vi "setup-reflux.vi"(8 "Reflux Ratio":dbl, 9 "Period (Seconds) in":dbl=5.0, 10 "Sampling Mode":T2(ring), 11 "delaytimes mS in":cluster{"low":dbl, "high":dbl}) -> (0 "Duty %":dbl, 1 "HIGH Cycle Time (Seconds)":dbl, 2 "LOW Cycle Time (Seconds)":dbl, 3 "delaytimes mS out":cluster{"low":dbl, "high":dbl}, 4 "Disabled":T1(ring), 6 "Period (Seconds) out":dbl)   [LabVIEW 2024]
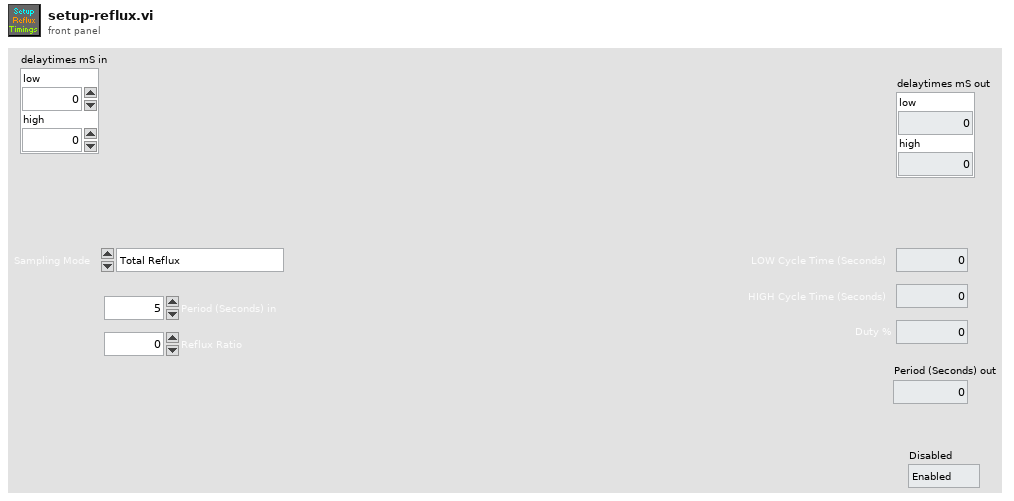
[diagram p1: front panel]
types:
  T1 = enum8{"Enabled", "Disabled", "Disabled and Grayed Out"}
  T2 = enum16{"Total Reflux", "Total Withdrawl", "Reflux Ratio"}
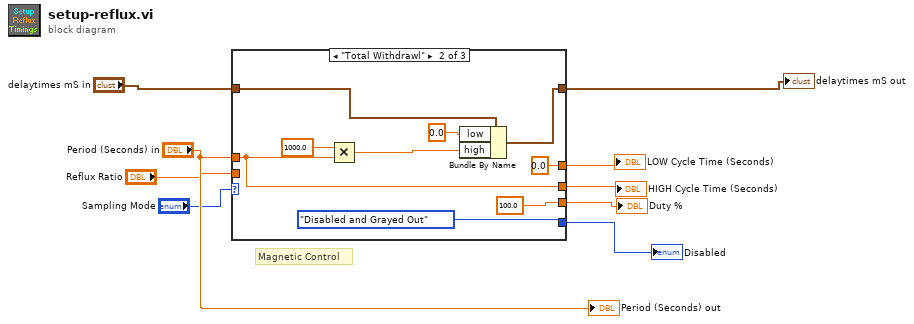
[diagram p0: block diagram]
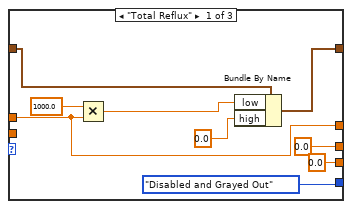
[diagram p2: hidden frame]
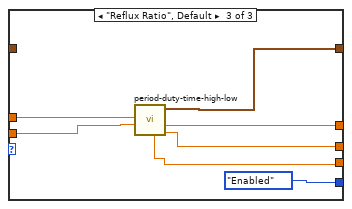
[diagram p3: hidden frame]
diagram:
  # "Magnetic Control"
  n1 = case shown="\"Total Withdrawl\"" "Sampling Mode" {
    tunnel: [w10 w26 w31] -> w4
    tunnel: "Period (Seconds) in" -> [w11 w24 w32]
    tunnel: "Reflux Ratio" -> [_ _ w33]
    tunnel: [w11 0.0 ("Time Low (Seconds)") w30] -> w5
    tunnel: [0.0 ("Time High (Seconds)") w24 w29] -> w6
    tunnel: [0.0 ("Duty %") 100.0 ("Duty %") w28] -> w7
    tunnel: [T1."Disabled and Grayed Out" ("Disabled") T1."Disabled and Grayed Out" ("Disabled") T1."Enabled" ("Disabled")] -> w1
    tunnel: "delaytimes mS in" -> [w18 w27 _]
    frame "Total Reflux" {
      n2 = Multiply(x=1000.0, y=w11) -> (x*y=w15:dbl)
      n3 = Bundle By Name(cluster=w18, "low"=w15, "high"=0.0) -> (w10:cluster{"low":dbl, "high":dbl})
    }
    frame "Total Withdrawl" {
      n4 = Multiply(x=1000.0, y=w24) -> (x*y=w22:dbl)
      n5 = Bundle By Name(cluster=w27, "low"=0.0, "high"=w22) -> (w26:cluster{"low":dbl, "high":dbl})
    }
    frame "Reflux Ratio", Default {
      n6 = call "period-duty-time-high-low.vi"("Duty Cycle"=w33, "Period (Seconds)"=w32) -> ("Time High (Seconds)"=w29:dbl, "Time Low (Seconds)"=w30:dbl, "delaytimes mS"=w31:cluster{"low":dbl, "high":dbl}, "Duty %"=w28:dbl)  [unwired: 6 in]
    }
  }
  "LOW Cycle Time (Seconds)" <- w5
  "HIGH Cycle Time (Seconds)" <- w6
  "Duty %" <- w7
  "delaytimes mS out" <- w4
  "Disabled" <- w1
  "Period (Seconds) out" <- "Period (Seconds) in"
